vi "Wait for waveform.vi"(5 "Time safe":bool=TRUE, 7 "Active":bool=TRUE, 8 "Error in":errorcluster, 9 "Sampling info":cluster{"Fs":dbl, "#s":dbl}={"Fs"=48000.0, "#s"=1000.0}, 11 "Samples":i32) -> (0 "Error out":errorcluster)   [LabVIEW 2019]
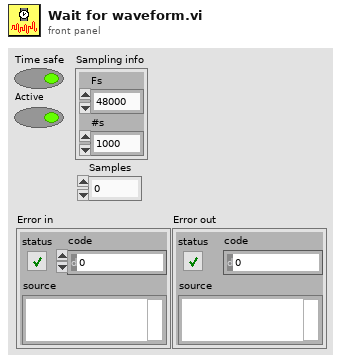
[diagram p1: front panel]
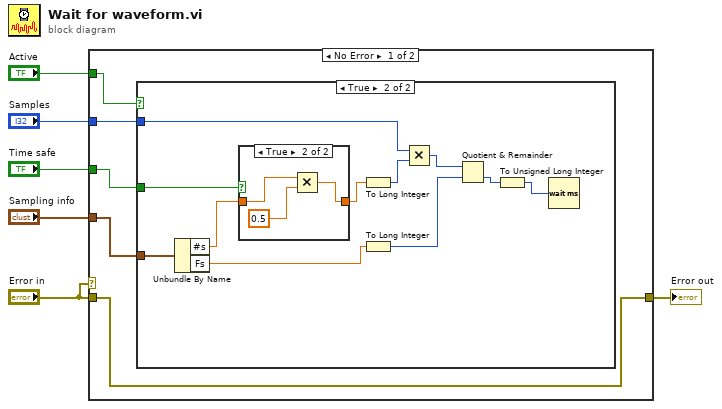
[diagram p0: block diagram]
diagram:
  n1 = case shown="No Error" "Error in" {
    tunnel: "Error in" -> [w8 w27]
    tunnel: [w8 w27] -> w5
    tunnel: "Time safe" -> [w11 _]
    tunnel: "Sampling info" -> [w10 _]
    tunnel: "Samples" -> [w9 _]
    tunnel: "Active" -> [w7 _]
    frame No Error {
      n2 = case shown="True" w7 {
        tunnel: w11 -> [_ w22]
        tunnel: w10 -> [_ w21]
        tunnel: w9 -> [_ w15]
        frame False {
        }
        frame True {
          n3 = Unbundle By Name(w21) -> ("#s"=w14:dbl, "Fs"=w13:dbl)
          n4 = case shown="True" w22 {
            tunnel: w14 -> [w23 w26]
            tunnel: [w23 w24] -> w18
            frame False {
            }
            frame True {
              n5 = Multiply(x=w26, y=0.5) -> (x*y=w24:dbl)
            }
          }
          n6 = To Long Integer(number=w18) -> (32bit integer=w16:i32)
          n7 = To Long Integer(number=w13) -> (32bit integer=w12:i32)
          n8 = Multiply(x=w15, y=w16) -> (x*y=w17:i32)
          n9 = Quotient & Remainder(x=w17, y=w12) -> (floor(x/y)=w19:i32)  [unwired: 1 out]
          n10 = To Unsigned Long Integer(number=w19) -> (unsigned 32bit integer=w20:u32)
          n11 = Wait (ms)(milliseconds to wait=w20) -> ()  [unwired: 1 out]
        }
      }
    }
    frame Error {
    }
  }
  "Error out" <- w5
